vi "DPTest-Simulate Response.vi"(0 "state":T1, 7 "freqs":dbl[](array[numeric]), 9 "L2":dbl) -> (8 "Stimulus out":dbl[][](array[numeric]))   [LabVIEW 2020]
uses:
  Typedefs/DP-Runtime State.ctl
  4d7382aa-da82-4a5e-b546-f30b57a76c94.vi
  90a97fba-9c1e-4e2a-8569-7bbd5edfb3ea.vi
  <vilib>/Analysis/NI_AALBase.lvlib
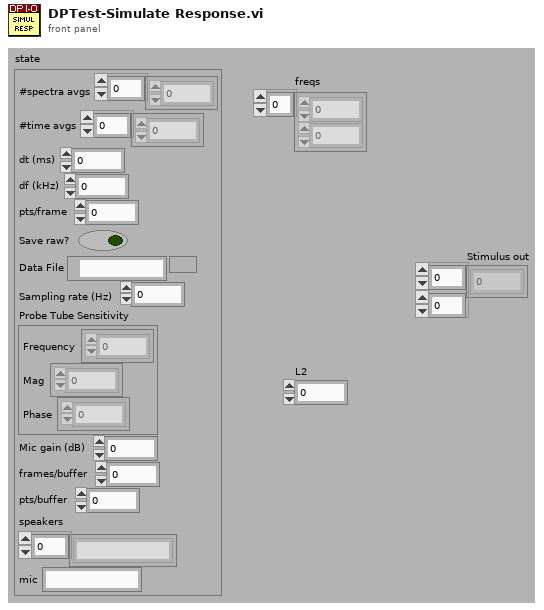
[diagram p1: front panel]
types:
  T1 = typedef "DP-Runtime State.ctl" = cluster{"#spectra avgs":i32[], "#time avgs":i32[], "dt (ms)":dbl, "df (kHz)":dbl, "pts/frame":i32, "Save raw?":bool, "Data File":path, "Sampling rate (Hz)":dbl, "Probe Tube Sensitivity":cluster{"Frequency":dbl[], "Mag":dbl[], "Phase":dbl[]}, "Mic gain (dB)":dbl, "frames/buffer":i32, "pts/buffer":i32, "speakers":string[], "mic":string}
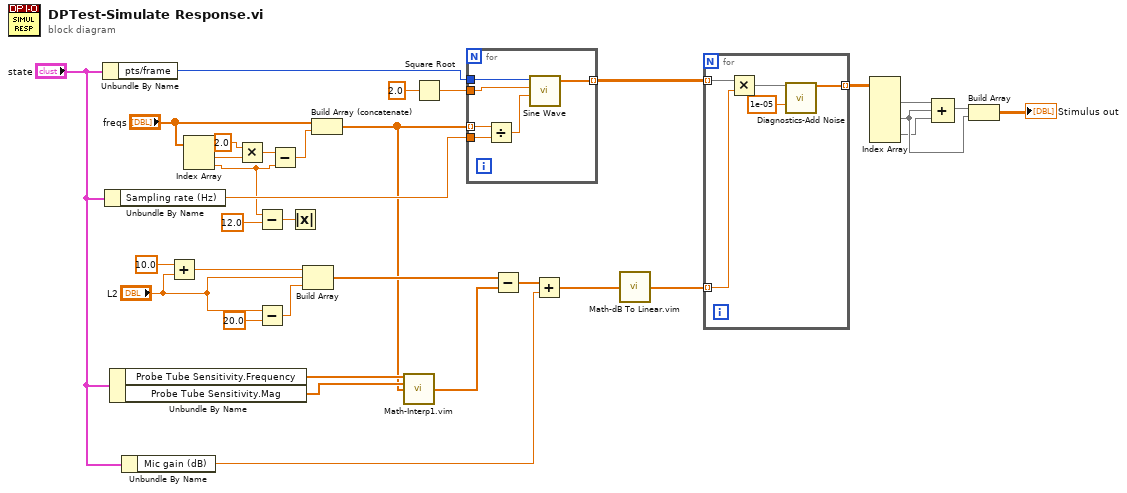
[diagram p0: block diagram]
diagram:
  n1 = Unbundle By Name("state") -> ("pts/frame"=w34:i32)
  n2 = Unbundle By Name("state") -> ("Sampling rate (Hz)"=w33:dbl)
  n3 = Unbundle By Name("state") -> ("Probe Tube Sensitivity.Frequency"=w19:dbl[], "Probe Tube Sensitivity.Mag"=w18:dbl[])
  n4 = Unbundle By Name("state") -> ("Mic gain (dB)"=w29:dbl)
  n5 = Add(x=10.0, y="L2") -> (x+y=w32:dbl)
  n6 = Index Array(array="freqs") -> (element #1=w13:dbl, element #2=w7:dbl)  [unwired: 2 in]
  n7 = Multiply(x=2.0, y=w13) -> (x*y=w11:dbl)
  n8 = Subtract(x=w7, y=12.0) -> (x-y=w5:dbl)
  n9 = Subtract(x="L2", y=20.0) -> (x-y=w2:dbl)
  n10 = Subtract(x=w11, y=w7) -> (x-y=w10:dbl)
  n11 = Absolute Value(x=w5) -> ()  [unwired: 1 out]
  n12 = Build Array(w32, "L2", w2) -> (w8:dbl[])
  n13 = Build Array (concatenate)("freqs", w10) -> (w1:dbl[])
  n14 = call "Math-Interp1.vim"("X"=w19, "Y"=w18, "U"=w1) -> ("V"=w31:dbl[])  [unwired: 12 in]
  n15 = Square Root(x=2.0) -> (sqrt(x)=w21:dbl)
  n16 = for {
    tunnel: w1 -> [w38] mode=indexing
    tunnel: w21 -> [w39]
    tunnel: w34 -> [w40]
    tunnel: w33 -> [w36]
    tunnel: [w35] -> w15 mode=indexing
    n17 = Divide(x=w38, y=w36) -> (x/y=w37:dbl)
    n18 = call <vilib>:"Sine Wave.vi"("samples"=w40, "amplitude"=w39, "frequency"=w37) -> ("sine wave"=w35:dbl[])  [unwired: 2 in, 2 out]
  }
  n19 = Subtract(x=w8, y=w31) -> (x-y=w30:dbl[])
  n20 = Add(x=w30, y=w29) -> (x+y=w28:dbl[])
  n21 = call "Math-dB To Linear.vim"("dB"=w28) -> ("linear"=w23:dbl[])
  n22 = for {
    tunnel: w15 -> [w45] mode=indexing
    tunnel: w23 -> [w44] mode=indexing
    tunnel: [w42] -> w27 mode=indexing
    n23 = Multiply(x=w45, y=w44) -> (x*y=w43:dbl[])
    n24 = call "Diagnostics-Add Noise.vi"("Signal"=w43, "Noise RMS"=1e-05) -> ("Signal + Noise"=w42:dbl[])  [unwired: 13 in]
  }
  n25 = Index Array(array=w27) -> (element #1=w26:dbl[], element #2=w24:dbl[], element #3=w16:dbl[])  [unwired: 6 in]
  n26 = Compound Arithmetic op=ADD(w26, w24, w16) -> (w25:dbl[])
  n27 = Build Array(w25, w24) -> (→"Stimulus out":dbl[][])
